vi "Open TCP IP Connection.vi"(8 "error in (no error)":errorcluster, 11 "Data Cluster in":T1={"Data Display"="", "FP Control Refs"={"Connect to Station Ref"=refnum, "Download Ref"=refnum, "Exit Button Ref"=refnum, "Start Date Refnum"=refnum, "End Date Refnum"=refnum, "Path"=refnum, "COM Port"="", "IP or Phone Ref"=refnum, "TCPIP ID"=refnum, "Reboot Refnum"=refnum, "Datafile Refnum"=refnum}, "FP Indicator Refs"={"Connected Refnum"=refnum, "Data Display Ref"=refnum, "Station ID Ref"=refnum}, "User Events"={"Stop"=refnum, "Update Display"=refnum}, "Message Queues"={"UI"=refnum, "ACQUISITION"=refnum, "PROCESSING"=refnum, "LOGGING"=refnum}, "IS IP?"=FALSE, "Downloading?"=FALSE, "DCP Version"=enum."XPert2", "Processing Loop State"=enum."Get Station  ID", "Username"=refnum, "Password"=refnum}) -> (0 "error out":errorcluster, 2 "Connected?":bool, 3 "Data Cluster out":T1={"Data Display"="", "FP Control Refs"={"Connect to Station Ref"=refnum, "Download Ref"=refnum, "Exit Button Ref"=refnum, "Start Date Refnum"=refnum, "End Date Refnum"=refnum, "Path"=refnum, "COM Port"="", "IP or Phone Ref"=refnum, "TCPIP ID"=refnum, "Reboot Refnum"=refnum, "Datafile Refnum"=refnum}, "FP Indicator Refs"={"Connected Refnum"=refnum, "Data Display Ref"=refnum, "Station ID Ref"=refnum}, "User Events"={"Stop"=refnum, "Update Display"=refnum}, "Message Queues"={"UI"=refnum, "ACQUISITION"=refnum, "PROCESSING"=refnum, "LOGGING"=refnum}, "IS IP?"=FALSE, "Downloading?"=FALSE, "DCP Version"=enum."XPert2", "Processing Loop State"=enum."Get Station  ID", "Username"=refnum, "Password"=refnum})   [LabVIEW 2018]
uses:
  Great Lakes Downloads/support/Message Queue/Enqueue Message (Single).vi
  Message Queue/Message Cluster.ctl
  Message Queue/GLDL Message Queue.lvlib
  Message Queue/All Message Queues.ctl
  controls/Connected Indicator.ctl
  controls/Output Indicator.ctl
  controls/Disconnect Control.ctl
  controls/Download Control.ctl
  controls/Exit Control.ctl
  controls/Date Control.ctl
  controls/IP Phone Number Control.ctl
  controls/GLDL UI Data.ctl
  controls/Station ID Indicator.ctl
  controls/Reboot Control.ctl
  controls/Processing Loop State.ctl
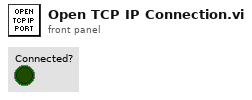
[diagram p1: front panel]
types:
  T1 = typedef "GLDL UI Data.ctl" = cluster{"Data Display":string, "FP Control Refs":cluster{"Connect to Station Ref":refnum<vi>, "Download Ref":refnum<vi>, "Exit Button Ref":refnum<vi>, "Start Date Refnum":refnum<vi>, "End Date Refnum":refnum<vi>, "Path":refnum<vi>, "COM Port":refnum<visa-resource-name>, "IP or Phone Ref":refnum<vi>, "TCPIP ID":refnum<k5>, "Reboot Refnum":refnum<vi>, "Datafile Refnum":refnum<file>}, "FP Indicator Refs":cluster{"Connected Refnum":refnum<vi>, "Data Display Ref":refnum<vi>, "Station ID Ref":refnum<vi>}, "User Events":cluster{"Stop":refnum<user-event>, "Update Display":refnum<user-event>}, "Message Queues":T2, "IS IP?":bool, "Downloading?":bool, "DCP Version":enum16{"XPert", "XPert2"}, "Processing Loop State":T3, "Username":refnum<vi>, "Password":refnum<vi>}
  T2 = typedef "GLDL Message Queue.lvlib/All Message Queues.ctl" = cluster{"UI":refnum<queue>, "ACQUISITION":refnum<queue>, "PROCESSING":refnum<queue>, "LOGGING":refnum<queue>}
  T3 = typedef "Processing Loop State.ctl" = enum16{"Get Station  ID", "Change Directory SD Card", "Change Directory Storage Card", "Downloading", "Idle in DL Directory"}
  T4 = enum16{"Standard", "Buffered", "CRLF", "Immediate"}
  T5 = typedef "IP Phone Number Control.ctl" = string
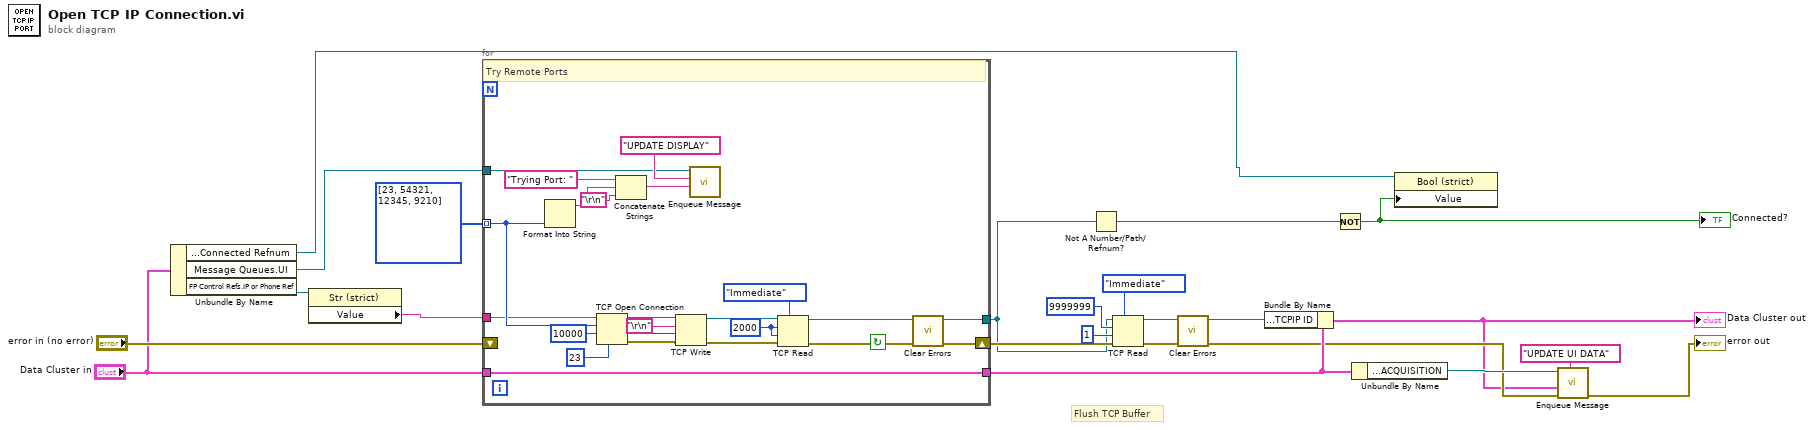
[diagram p0: block diagram]
diagram:
  # "Flush TCP Buffer"
  n1 = Unbundle By Name("Data Cluster in") -> ("FP Indicator Refs.Connected Refnum"=w9:refnum<vi>, "Message Queues.UI"=w15:refnum<queue>, "FP Control Refs.IP or Phone Ref"=w16:refnum<vi>)
  n2 = property class="Str (strict)"(reference=w16) -> ("Value"=w14:T5)  [unwired: 1 in, 2 out]
  n3 = for {
    tunnel: u16[] [23, 54321, 12345, 9210] ("remote port or service name") -> [w29] mode=indexing
    tunnel: w15 -> [w30]
    tunnel: w14 -> [w28]
    shift-right: [w26] -> w12
    shift-left: "error in (no error)" -> [_]
    tunnel: "Data Cluster in" -> [w24]
    tunnel: [w25] -> w10
    tunnel: [w24] -> w5
    stop <- w27 continue-if-true
    w32 = 2000 ("timeout ms (25000)")
    w33 = 10000 ("timeout ms (60000)")
    # "Try Remote Ports"
    n4 = Format Into String(w29) -> (resulting string=w43:string)  [unwired: 3 in, 1 out]
    n5 = TCP Open Connection(address=w28, remote port or service name=w29, timeout ms (60000)=w33, local port=u16 23 ("local port (0)")) -> (connection ID=w34:refnum<k5>, error out=w37:errorcluster)  [unwired: 1 in]
    n6 = Concatenate Strings("Trying Port: " ("Message"), w43, "\r\n") -> (w39:string)
    n7 = TCP Write(connection ID=w34, data in="\r\n", error in (no error)=w37, 9:w33) -> (connection ID out=w35:refnum<k5>, error out=w36:errorcluster)  [unwired: 1 out]
    n8 = call-poly "Enqueue Message.vi"("Message Data"=w39, "Message"="UPDATE DISPLAY", "Message Queue"=w30) -> ()  [unwired: 7 in, 2 out]
    n9 = TCP Read(connection ID=w35, bytes to read=w32, error in (no error)=w36, 7:T4."Immediate" ("mode (standard)"), 9:w32) -> (connection ID out=w25:refnum<k5>, error out=w27:errorcluster)  [unwired: 1 out]
    n10 = call <vilib>:"Clear Errors.vi"("error in (no error)"=w27) -> ("error out"=w26:errorcluster)  [unwired: 5 in, 1 out]
  }
  n11 = Not A Number/Path/Refnum?(number/path/refnum=w10) -> (NaN/Path/Refnum?=w8:bool)
  n12 = TCP Read(connection ID=w10, bytes to read=9999999 ("timeout ms (25000)"), error in (no error)=w12, 7:T4."Immediate" ("mode (standard)"), 9:1 ("timeout ms (25000)")) -> (connection ID out=w19:refnum<k5>, error out=w18:errorcluster)  [unwired: 1 out]
  n13 = call <vilib>:"Clear Errors.vi"("error in (no error)"=w18) -> ("error out"=w3:errorcluster)  [unwired: 5 in, 1 out]
  n14 = Bundle By Name(cluster=w5, "FP Control Refs.TCPIP ID"=w19) -> (w2:T1)
  "Data Cluster out" <- w2
  n15 = Not(x=w8) -> (.not. x?=w7:bool)
  "Connected?" <- w7
  n16 = Unbundle By Name(w5) -> ("Message Queues.ACQUISITION"=w4:refnum<queue>)
  n17 = property class="Bool (strict)"(reference=w9, "Value"=w7) -> ()  [unwired: 1 in, 2 out]
  n18 = call-poly "Enqueue Message.vi"("error in (no error)"=w3, "Message Data"=w2, "Message"="UPDATE UI DATA", "Message Queue"=w4) -> ("error out"=→"error out":errorcluster)  [unwired: 6 in, 1 out]
